vi "Convert Voltage to Angle.vi"(10 "Inclinometer output (V)":dbl=0.5 min=0.5 max=4.5) -> (2 "Angle":dbl)   [LabVIEW 2018]
panel:
  # "Control Properties>>Data Entry set to be between 0.5 and 4.5.\nCoerce if value is outside of limits."
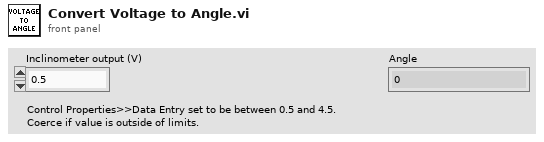
[diagram p1: front panel]
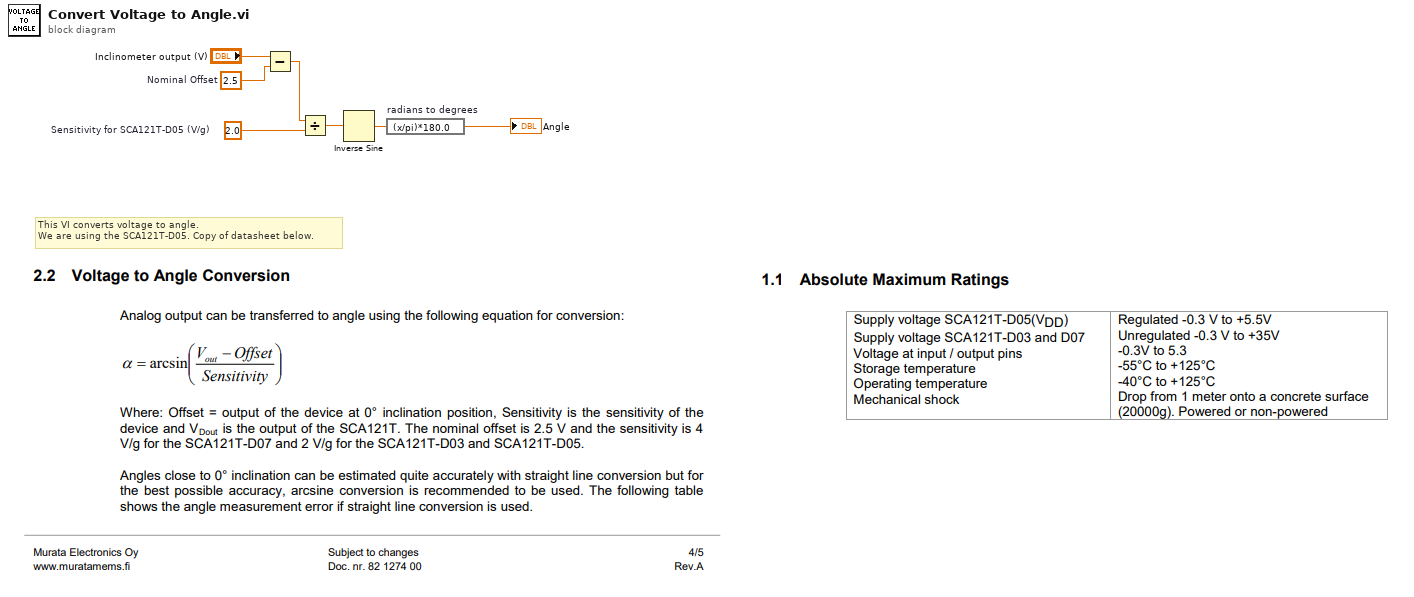
[diagram p0: block diagram]
diagram:
  w3 = 2.5  # Nominal Offset
  w6 = 2.0  # Sensitivity for SCA121T-D05 (V/g)
  # "This VI converts voltage to angle.\nWe are using the SCA121T-D05. Copy of datasheet below."
  n1 = Subtract(x="Inclinometer output (V)", y=w3) -> (x-y=w5:dbl)
  n2 = Divide(x=w5, y=w6) -> (x/y=w7:dbl)
  n3 = Inverse Sine(1:w7) -> (0:w2:dbl)
  n4 = expression code="(x/pi)*180.0" "radians to degrees"(w2) -> (→"Angle":dbl)
